vi "UserAuthentication.vi"(8 "error in (no error)":errorcluster, 9 "UserID":string, 10 "Password":string, 11 "path":path) -> (0 "error out":errorcluster, 2 "Boolean":bool, 3 "UserName":string)   [LabVIEW 2018]
uses:
  <vilib>/Utility/config.llb/Read Key (String).vi
  <vilib>/Utility/config.llb/NI_LVConfig.lvlib
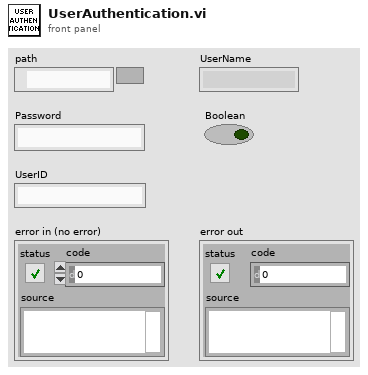
[diagram p1: front panel]
types:
  T1 = typedef "NI_LVConfig.lvlib/Config Data RefNum.ctl" = refnum<k1>
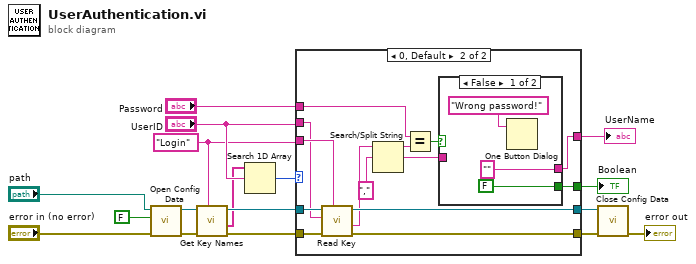
[diagram p0: block diagram]
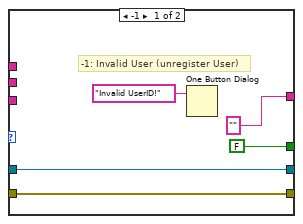
[diagram p2: hidden frame]
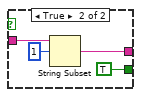
[diagram p3: hidden frame]
diagram:
  w7 = "Login" ("section")
  n1 = call <vilib>:"Open Config Data.vi"("error in (no error)"="error in (no error)", "create file if necessary (T)"=FALSE, "configuration file path"="path") -> ("error out"=w3:errorcluster, "refnum"=w4:T1)  [unwired: 6 in, 1 out]
  n2 = call <vilib>:"Get Key Names.vi"("section"=w7, "error in (no error)"=w3, "refnum"=w4) -> ("error out"=w8:errorcluster, "key names"=w5:string[], "refnum out"=w6:T1)  [unwired: 5 in, 1 out]
  n3 = Search 1D Array(1D array=w5, element="UserID") -> (index of element=w1:i32)  [unwired: 1 in]
  n4 = case shown="0, Default" w1 {
    tunnel: w6 -> [w21 w36]
    tunnel: w7 -> [_ w35]
    tunnel: "UserID" -> [_ w34]
    tunnel: w8 -> [w20 w33]
    tunnel: "Password" -> [_ w32]
    tunnel: [w20 w29] -> w9
    tunnel: [w21 w30] -> w10
    tunnel: ["" ("value") w24] -> w15
    tunnel: [FALSE ("Success") w23] -> w17
    frame -1 {
      # "-1: Invalid User (unregister User)"
      n5 = One Button Dialog(message="Invalid UserID!") -> ()  [unwired: 1 in, 1 out]
    }
    frame 0, Default {
      n6 = call-poly <vilib>:"Read Key.vi"("section"=w35, "error in (no error)"=w33, "key"=w34, "refnum"=w36) -> ("error out"=w29:errorcluster, "value"=w28:string, "refnum out"=w30:T1)  [unwired: 4 in, 1 out]
      n7 = Search/Split String(string=w28, search string/char (-)=",") -> (substring before match=w26:string, match + rest of string=w25:string)  [unwired: 1 in, 1 out]
      n8 = Equal?(x=w32, y=w26) -> (x = y?=w31:bool)
      n9 = case shown="False" w31 {
        tunnel: w25 -> [_ w43]
        tunnel: ["" ("value") w41] -> w24
        tunnel: [FALSE ("Success") TRUE ("Boolean")] -> w23
        frame False {
          n10 = One Button Dialog(message="Wrong password!") -> ()  [unwired: 1 in, 1 out]
        }
        frame True {
          n11 = String Subset(string=w43, offset (0)=1) -> (substring=w41:string)  [unwired: 1 in]
        }
      }
    }
  }
  "Boolean" <- w17
  "UserName" <- w15
  n12 = call <vilib>:"Close Config Data.vi"("error in (no error)"=w9, "refnum"=w10) -> ("error out"=→"error out":errorcluster)  [unwired: 8 in, 1 out]
